vi "Close Spreadsheet.vi"(8 "error in (no error)":errorcluster, 11 "Excel XML in":refnum<class "Excel XML.lvclass">) -> (0 "error out":errorcluster, 3 "Excel XML out":refnum<class "Excel XML.lvclass">)   [LabVIEW 2013, in "Excel XML.lvclass"]
uses:
  Excel XML.lvclass
  Spreadsheet.lvclass
  Excel XML.lvclass/Excel XML.ctl
  C:/PhaeronGit/LVNPOI/Resources/NPOI 2.1.1 dotnet4/NPOI.OOXML.dll
  Resources/NPOI 2.1.1 dotnet4/NPOI.OOXML.dll
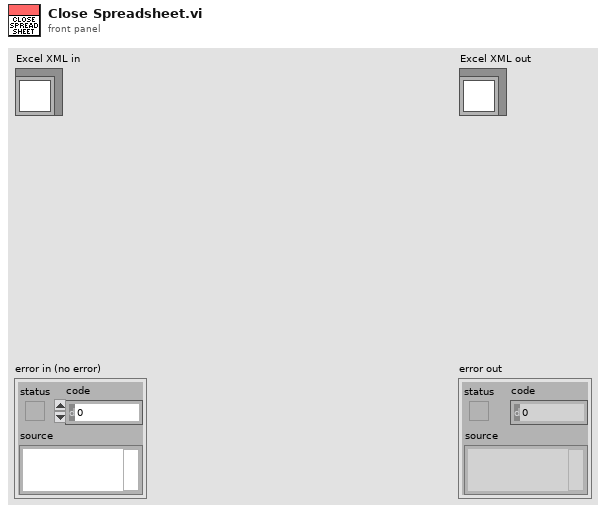
[diagram p1: front panel]
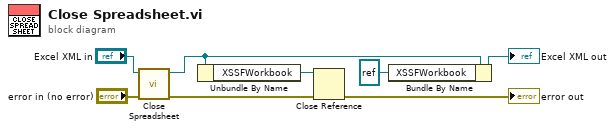
[diagram p0: block diagram]
diagram:
  n1 = call-parent "Close Spreadsheet.vi"("error in (no error)"="error in (no error)", "Spreadsheet in"="Excel XML in") -> ("error out"=w6:errorcluster, "Spreadsheet out"=w4:refnum<class "Excel XML.lvclass">)  [unwired: 8 in]
  n2 = Unbundle By Name(w4) -> ("XSSFWorkbook"=w3:refnum<k24>)
  n3 = Close Reference(reference=w3, error in (no error)=w6) -> (error out=→"error out":errorcluster)
  n4 = Bundle By Name(cluster=w4, "XSSFWorkbook"=refnum<k24> refnum) -> (→"Excel XML out":refnum<class "Excel XML.lvclass">)
